vi "Create Missing Folder.vi"(8 "error in":errorcluster, 11 "path":path) -> (0 "error out":errorcluster, 2 "path existed?":bool, 3 "path dup":path)   [LabVIEW 2016]
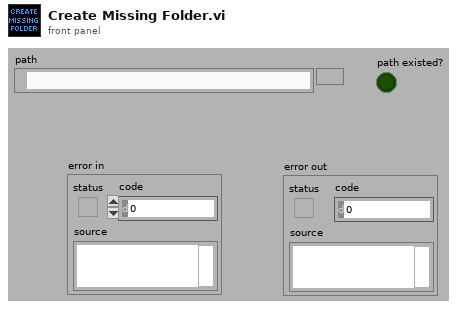
[diagram p1: front panel]
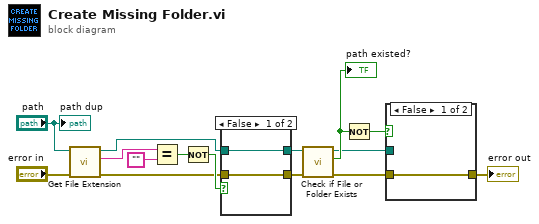
[diagram p0: block diagram]
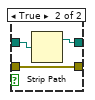
[diagram p2: hidden frame]
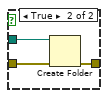
[diagram p3: hidden frame]
diagram:
  n1 = call <vilib>:"Get File Extension.vi"("error in (no error)"="error in", "file"="path") -> ("error out"=w4:errorcluster, "lowercase file extension"=w2:string, "dup file"=w3:path)  [unwired: 5 in, 2 out]
  n2 = Equal?(x=w2, y="") -> (x = y?=w1:bool)
  n3 = Not(x=w1) -> (.not. x?=w11:bool)
  n4 = case shown="False" w11 {
    tunnel: w3 -> [w17 w20]
    tunnel: [w17 w19] -> w10
    tunnel: w4 -> [w16 w18]
    tunnel: [w16 w18] -> w9
    frame False {
    }
    frame True {
      n5 = Strip Path(path=w20) -> (stripped path=w19:path)  [unwired: 1 out]
    }
  }
  n6 = call <vilib>:"Check if File or Folder Exists.vi"("error in (no error)"=w9, "path"=w10) -> ("error out"=w13:errorcluster, "file or folder exists?"=w15:bool, "dup path"=w14:path)  [unwired: 7 in]
  "path existed?" <- w15
  n7 = Not(x=w15) -> (.not. x?=w12:bool)
  n8 = case shown="False" w12 {
    tunnel: w14 -> [_ w24]
    tunnel: w13 -> [w21 w23]
    tunnel: [w21 w22] -> w8
    frame False {
    }
    frame True {
      n9 = Create Folder(path (use dialog)=w24, error in=w23) -> (error out=w22:errorcluster)  [unwired: 1 in, 2 out]
    }
  }
  "error out" <- w8
  "path dup" <- "path"
